vi "getModelInfo.vi"(0 "VISA resource name":refnum<visa-resource-name>, 11 "error in (no error)":errorcluster) -> (4 "VISA resource name out":refnum<visa-resource-name>, 6 "Model Names":string[](array[string]), 8 "Microstep Sizes":dbl[](array[numeric]), 10 "Device Number & Axis":string[](array[string]), 14 "Motion Type":string[](array[string]), 15 "error out":errorcluster)   [LabVIEW 2020, in "ZaberASeries.lvclass"]
uses:
  ZaberASeries.lvclass
  Zaber A Series.lvlib
panel:
  out "Axis Counts by Device":i32[][](array[numeric])
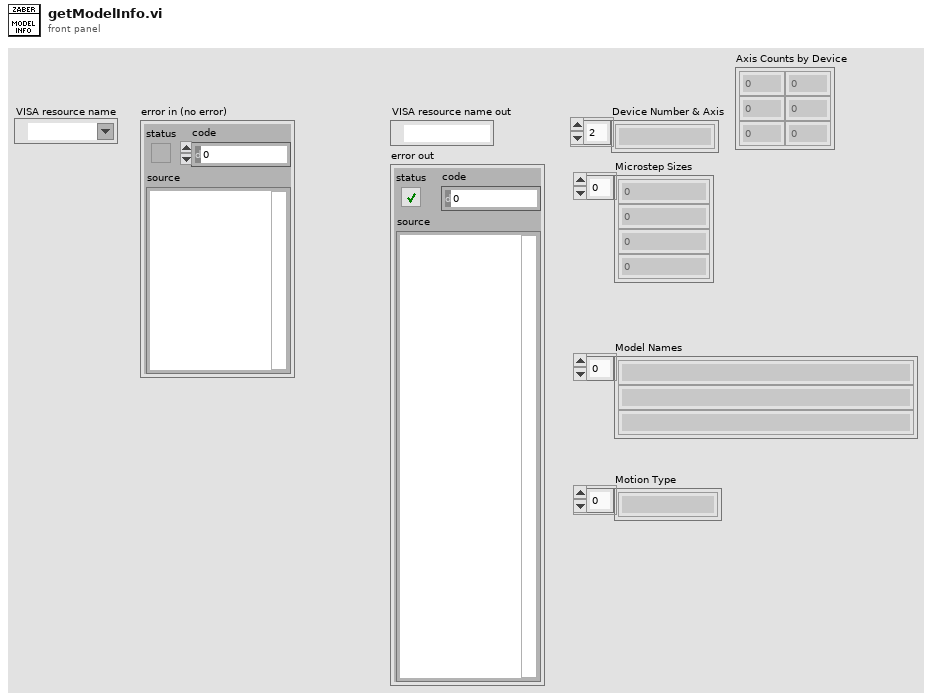
[diagram p1: front panel]
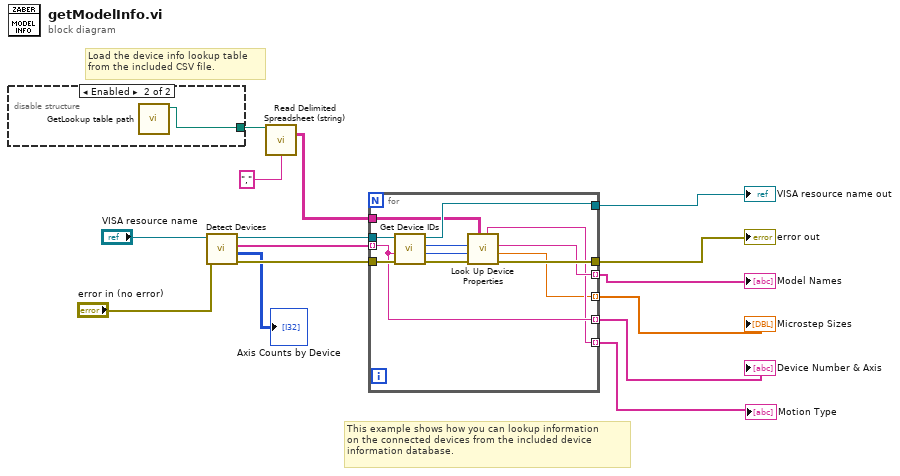
[diagram p0: block diagram]
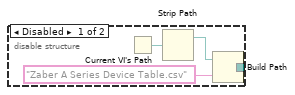
[diagram p2: hidden frame]
diagram:
  # "Load the device info lookup table\nfrom the included CSV file."
  # "This example shows how you can lookup information\non the connected devices from the included device \ninformation database."
  n1 = disable-structure shown="Enabled" {
    disable-tunnel: [w16 w20] -> w8
    frame Disabled {
      n2 = Current VI's Path() -> (path=w18:path)
      n3 = Strip Path(path=w18) -> (stripped path=w19:path)  [unwired: 1 out]
      n4 = Build Path(base path=w19, name or relative path="Zaber A Series Device Table.csv") -> (appended path=w16:path)
    }
    frame Enabled {
      n5 = call "GetLookup table path.vi"() -> ("device table path"=w20:path)  [unwired: 11 in]
    }
  }
  n6 = call "Detect Devices.vi"("error in (no error)"="error in (no error)", "VISA resource name"="VISA resource name") -> ("error out"=w10:errorcluster, "Axis Counts by Device"=→"Axis Counts by Device":i32[][], "Connected Devices and Axes"=w11:string[], "VISA resource name out"=w9:refnum<visa-resource-name>)  [unwired: 6 in]
  n7 = call "Read Delimited Spreadsheet (string).vi"("file path (dialog if empty)"=w8, "delimiter (\\t)"="," ("delimiter (\\t)")) -> ("all rows"=w6:string[][])  [unwired: 8 in, 5 out]
  n8 = for {
    tunnel: w9 -> [w32]
    tunnel: w10 -> [w31]
    tunnel: [w27] -> w2
    tunnel: w11 -> [w26] mode=indexing
    tunnel: [w26] -> w12 mode=indexing
    tunnel: [w25] -> w13 mode=indexing
    tunnel: [w21] -> w14 mode=indexing
    tunnel: [w24] -> w15 mode=indexing
    tunnel: [w23] -> w3
    tunnel: w6 -> [w22]
    n9 = call "Get Device IDs.vi"("error in (no error)"=w31, "Device and Axis"=w26, "VISA resource name"=w32) -> ("error out"=w28:errorcluster, "Peripheral ID"=w29:i32, "Device ID"=w30:i32, "VISA resource name out"=w23:refnum<visa-resource-name>)  [unwired: 5 in]
    n10 = call "Look Up Device Properties.vi"("Lookup Table"=w22, "error in (no error)"=w28, "Peripheral ID (0)"=w29, "Device ID"=w30) -> ("error out"=w27:errorcluster, "Microstep Size"=w21:dbl, "Device Name"=w25:string, "Motion Type"=w24:string)  [unwired: 4 in]
  }
  "VISA resource name out" <- w3
  "error out" <- w2
  "Model Names" <- w13
  "Microstep Sizes" <- w14
  "Device Number & Axis" <- w12
  "Motion Type" <- w15
